vi "picture.get.vi"(8 "error in":errorcluster, 11 "midi-ui in":refnum<class "midi-ui.lvclass">) -> (0 "error out":errorcluster, 3 "midi-ui out":refnum<class "midi-ui.lvclass">)   [LabVIEW 2020, in "midi-ui.lvclass"]
uses:
  midi-ui.lvclass
  midi-ui.lvclass/midi-ui.ctl
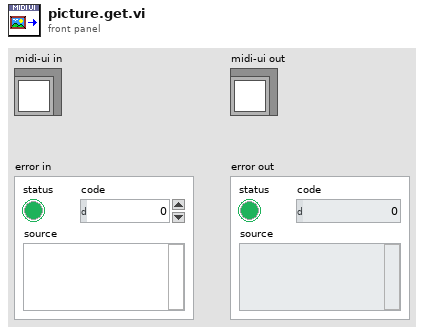
[diagram p1: front panel]
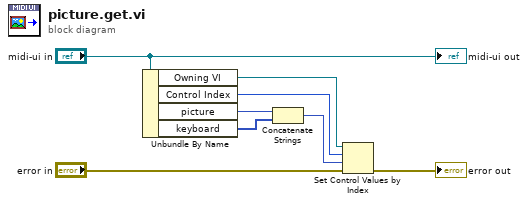
[diagram p0: block diagram]
diagram:
  n1 = Unbundle By Name("midi-ui in") -> ("Owning VI"=w5:refnum<vi>, "Control Index"=w8:i32, "picture"=w2:picture, "keyboard"=w4:picture[])
  n2 = Concatenate Strings(w2, w4) -> (w3:picture)
  n3 = Set Control Values by Index(0:w5, 1:w8, 2:w3, 3:"error in") -> (11:→"error out":errorcluster)
  "midi-ui out" <- "midi-ui in"
